vi "Motion_Clear Errors.vi"(8 "error in (no error)":errorcluster, 11 "TCP Connection Refnum in":refnum<k5>) -> (0 "error out":errorcluster, 3 "TCP Connection Refnum (dup)":refnum<k5>)   [LabVIEW 2010]
uses:
  <vilib>/NI Modbus.llb/MB Ethernet Master Query Write Single Coil (poly).vi
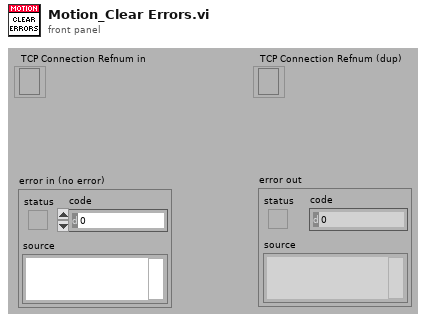
[diagram p1: front panel]
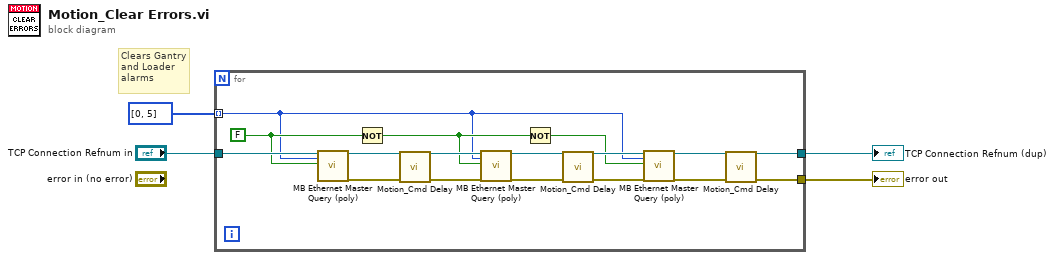
[diagram p0: block diagram]
diagram:
  # "Clears Gantry and Loader alarms"
  n1 = for {
    tunnel: [w21] -> w4
    tunnel: "TCP Connection Refnum in" -> [w20]
    tunnel: [w19] -> w2
    tunnel: u16[] [0, 5] -> [w5] mode=indexing
    w8 = FALSE
    n2 = call-poly <vilib>:"MB Ethernet Master Query (poly).vi"("TCP Connection Refnum in"=w20, "Address"=w5, "Coil"=w8) -> ("TCP Connection Refnum (dup)"=w18:refnum<k5>, "error out"=w17:errorcluster)  [unwired: 14 in, 1 out]
    n3 = Not(x=w8) -> (.not. x?=w7:bool)
    n4 = call "Motion_Cmd Delay.vi"("error in"=w17, "TCP Connection Refnum"=w18) -> ("error out"=w16:errorcluster, "TCP Connection Refnum (dup)"=w15:refnum<k5>)  [unwired: 8 in]
    n5 = call-poly <vilib>:"MB Ethernet Master Query (poly).vi"("TCP Connection Refnum in"=w15, "Address"=w5, "Coil"=w7, "error in"=w16) -> ("TCP Connection Refnum (dup)"=w9:refnum<k5>, "error out"=w14:errorcluster)  [unwired: 13 in, 1 out]
    n6 = Not(x=w7) -> (.not. x?=w6:bool)
    n7 = call "Motion_Cmd Delay.vi"("error in"=w14, "TCP Connection Refnum"=w9) -> ("error out"=w12:errorcluster, "TCP Connection Refnum (dup)"=w13:refnum<k5>)  [unwired: 8 in]
    n8 = call-poly <vilib>:"MB Ethernet Master Query (poly).vi"("TCP Connection Refnum in"=w13, "Address"=w5, "Coil"=w6, "error in"=w12) -> ("TCP Connection Refnum (dup)"=w11:refnum<k5>, "error out"=w10:errorcluster)  [unwired: 13 in, 1 out]
    n9 = call "Motion_Cmd Delay.vi"("error in"=w10, "TCP Connection Refnum"=w11) -> ("error out"=w21:errorcluster, "TCP Connection Refnum (dup)"=w19:refnum<k5>)  [unwired: 8 in]
  }
  "error out" <- w4
  "TCP Connection Refnum (dup)" <- w2
